vi "Modified Packages.vi"(7 "error in":errorcluster, 10 "Pagckages in":T2) -> (0 "error out":errorcluster, 2 "Cancel?":bool, 3 "Modified Packages":T1)   [LabVIEW 2019, in "GUI.lvlib"]
uses:
  GUI.lvlib
  527ef637-5418-40b0-a291-c1c2b8189254.vi
panel:
  in  "Cancel":bool
  in  "OK":bool
  in  "Packages":T1
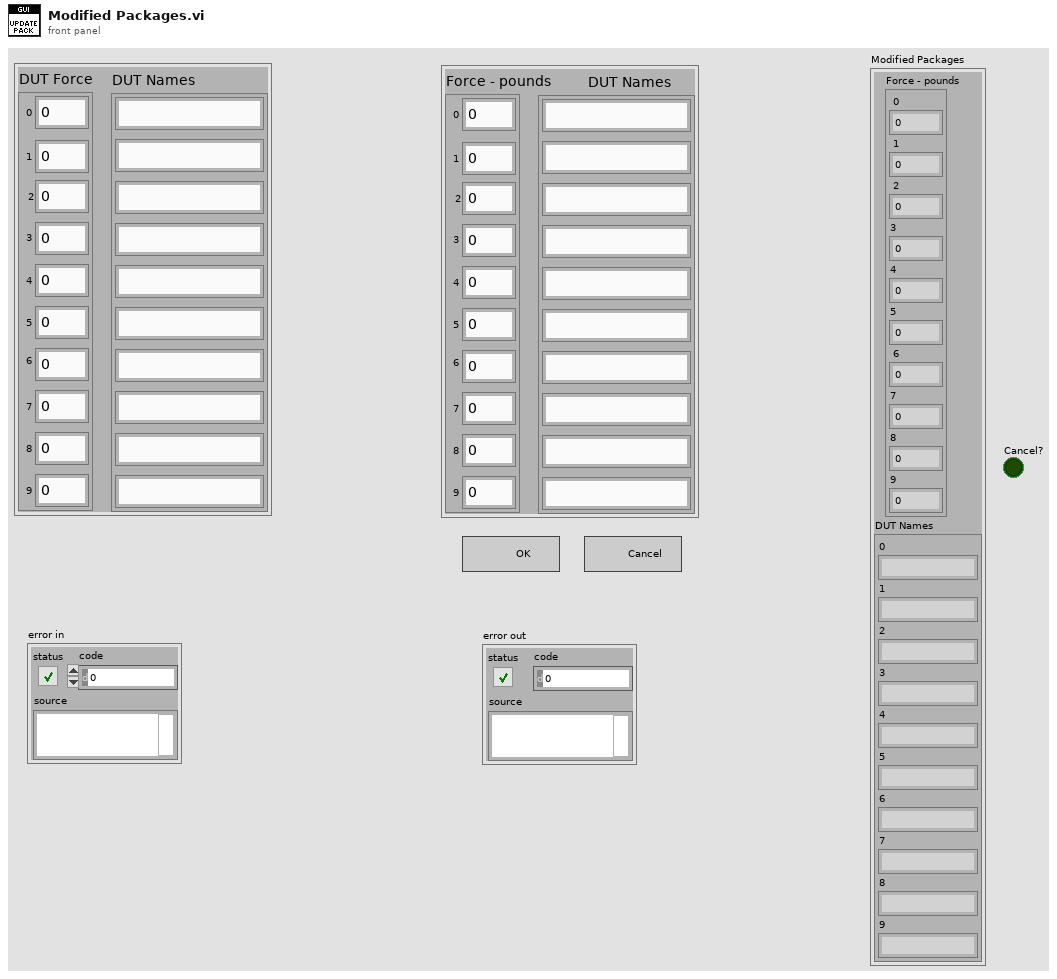
[diagram p1: front panel]
types:
  T1 = cluster{"Force - pounds":cluster{" 0":u32, " 1":u32, " 2":u32, "3":u32, "4":u32, "5":u32, " 6":u32, "7":u32, "8":u32, "9":u32}, "DUT Names":cluster{"0":string, "1":string, "2":string, "3":string, "4":string, "5":string, "6":string, "7":string, "8":string, "9":string}}
  T2 = cluster{"DUT Force":cluster{" 0":u32, " 1":u32, " 2":u32, "3":u32, "4":u32, "5":u32, " 6":u32, "7":u32, "8":u32, "9":u32}, "DUT Names":cluster{"0":string, "1":string, "2":string, "3":string, "4":string, "5":string, "6":string, "7":string, "8":string, "9":string}}
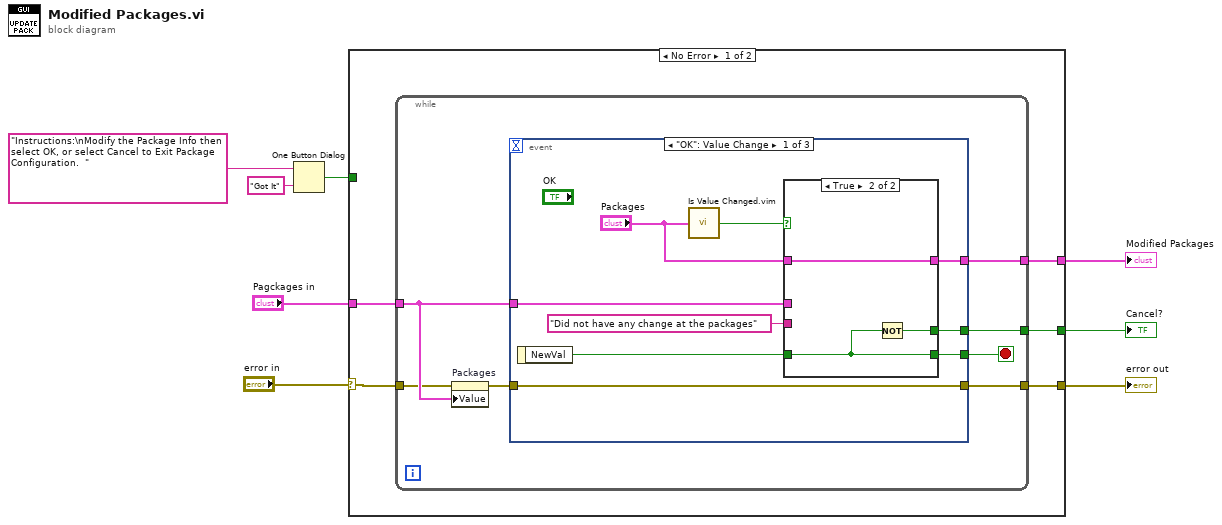
[diagram p0: block diagram]
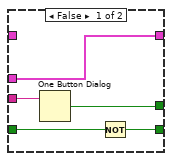
[diagram p2: hidden frame]
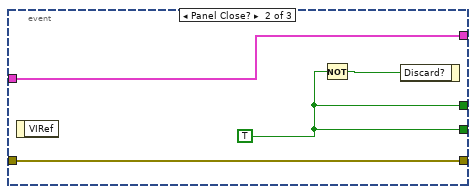
[diagram p3: hidden frame]
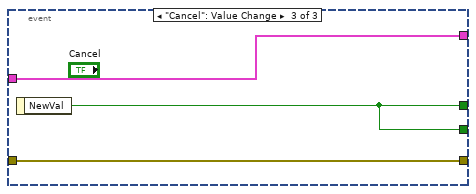
[diagram p4: hidden frame]
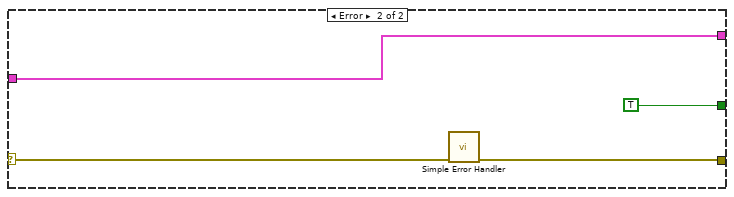
[diagram p5: hidden frame]
diagram:
  n1 = One Button Dialog(message="Instructions:\nModify the Package Info then select OK, or select Cancel to Exit Package Configuration.  ", button name ("OK")="Got It") -> (true=w4:bool)
  n2 = case shown="No Error" "error in" {
    selector: "error in" -> [w11 w48]
    tunnel: [w9 w47] -> w7
    tunnel: w4 -> [_ _]
    tunnel: "Pagckages in" -> [w13 w46]
    tunnel: [w12 TRUE ("NewVal")] -> w2
    tunnel: [w10 w46] -> w1
    frame No Error {
      n3 = while {
        tunnel: w13 -> [w19]
        tunnel: [w20] -> w12
        tunnel: w11 -> [w18]
        tunnel: [w15] -> w10
        tunnel: [w14] -> w9
        stop <- w16 stop-if-true
        n4 = property on="Packages" class="Clust (strict)"(error in=w18, "Value"=w19) -> (error out=w17:errorcluster)  [unwired: 1 in, 1 out]
        n5 = event shown="[0] \"OK\": Value Change" {
          selector: _ -> [_ _ _]
          dyn-events: _ -> [_ _ _]
          timeout: _ -> [_ _ _]
          tunnel: w19 -> [w27 w38 w42]
          tunnel: [w26 w38 w42] -> w15
          tunnel: [w22 w40 w44] -> w20
          tunnel: w17 -> [w29 w39 w43]
          tunnel: [w24 w40 w44] -> w16
          tunnel: [w29 w39 w43] -> w14
          event "OK": Value Change {
            n6 = event-data() -> ("NewVal"=w23:bool)  [unwired: 1 in]
            n7 = call "Is Value Changed.vim"("value"="Packages") -> ("changed or first call?"=w28:bool)
            n8 = case shown="True" w28 {
              tunnel: w27 -> [w34 _]
              tunnel: [w34 w37] -> w26
              tunnel: "Packages" -> [_ w37]
              tunnel: [w30 w36] -> w24
              tunnel: w23 -> [w31 w36]
              tunnel: [w32 w35] -> w22
              tunnel: "Did not have any change at the packages" ("message") -> [w33 _]
              frame False {
                n9 = One Button Dialog(message=w33) -> (true=w32:bool)  [unwired: 1 in]
                n10 = Not(x=w31) -> (.not. x?=w30:bool)
              }
              frame True {
                n11 = Not(x=w36) -> (.not. x?=w35:bool)
              }
            }
          }
          event Panel Close? {
            w40 = TRUE ("NewVal")
            n12 = event-data() -> ()  [unwired: 1 in, 1 out]
            n13 = Not(x=w40) -> (.not. x?=w41:bool)
            n14 = event-data("Discard?"=w41) -> ()  [unwired: 1 in, 1 out]
          }
          event "Cancel": Value Change {
            n15 = event-data() -> ("NewVal"=w44:bool)  [unwired: 1 in]
          }
        }
      }
    }
    frame Error {
      n16 = call <vilib>:"Simple Error Handler.vi"("error in (no error)"=w48) -> ("error out"=w47:errorcluster)  [unwired: 4 in, 4 out]
    }
  }
  "error out" <- w7
  "Cancel?" <- w2
  "Modified Packages" <- w1
